vi "Read Timing Grps.vi"(8 "error in (no error)":errorcluster, 11 "Chassis Cfg":refnum<class "ChassisCfg.lvclass">) -> (0 "error out":errorcluster, 2 "Timing Grps":refnum<class "TimingGrp.lvclass">[](array[class]), 3 "Chassis Cfg":refnum<class "ChassisCfg.lvclass">)   [LabVIEW 2018, in "Configuration Grandmaster.lvlib" / "ChassisCfg.lvclass"]
uses:
  ChassisCfg.lvclass
  Class Timing Group/TimingGrp.lvclass
  ChassisCfg.lvclass/ChassisCfg.ctl
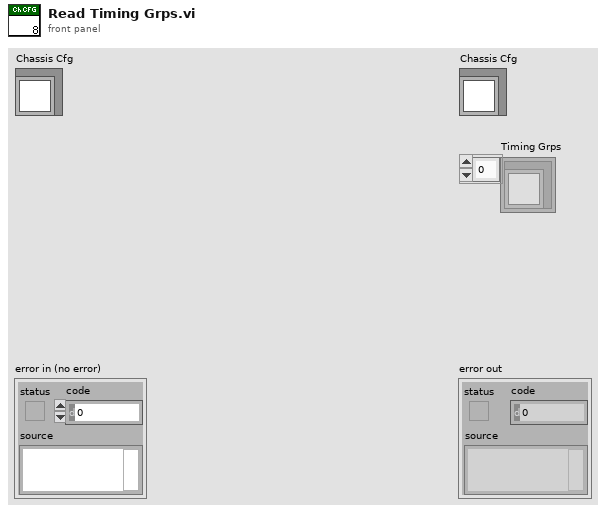
[diagram p1: front panel]
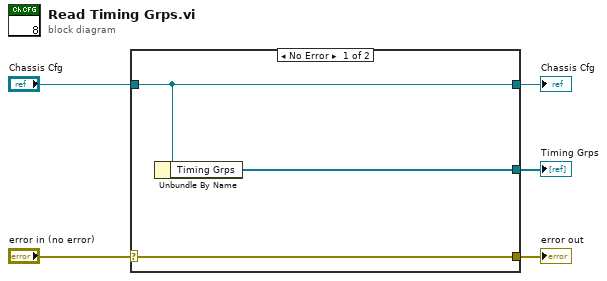
[diagram p0: block diagram]
diagram:
  n1 = case shown="No Error" "error in (no error)" {
    selector: "error in (no error)" -> [w8 w9]
    tunnel: [w8 w9] -> w4
    tunnel: [w7 w10] -> w2
    tunnel: "Chassis Cfg" -> [w7 w10]
    tunnel: [w6 _] -> w1
    frame No Error {
      n2 = Unbundle By Name(w7) -> ("Timing Grps"=w6:refnum<class "TimingGrp.lvclass">[])
    }
    frame Error {
    }
  }
  "error out" <- w4
  "Chassis Cfg" <- w2
  "Timing Grps" <- w1
